vi "StudentScope - Calculate Cursor Values.vi"(5 "Scope graph":refnum<vi>, 6 "C2 Select":u32, 7 "C1 Select":u32, 8 "Array":dbl[][](array[numeric]), 9 "Rate":dbl) -> (0 "C2 Voltage":string, 1 "dV":string, 2 "C1 Voltage":string, 3 "dT":string)   [LabVIEW 2015]
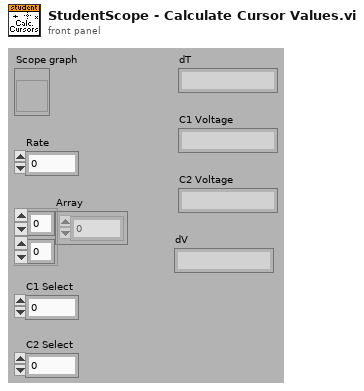
[diagram p1: front panel]
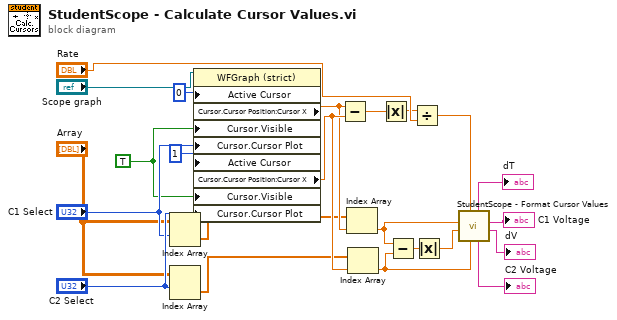
[diagram p0: block diagram]
diagram:
  w17 = TRUE ("Cursor.Visible")
  n1 = Index Array(array="Array", index (row)="C1 Select") -> (element=w11:dbl[])  [unwired: 1 in]
  n2 = Index Array(array="Array", index (row)="C2 Select") -> (element=w12:dbl[])  [unwired: 1 in]
  n3 = property class="WFGraph (strict)"(reference="Scope graph", "Active Cursor"=u32 0, "Cursor.Visible"=w17, "Cursor.Cursor Plot"="C1 Select", "Active Cursor"=u32 1, "Cursor.Visible"=w17, "Cursor.Cursor Plot"="C2 Select") -> ("Cursor.Cursor Position:Cursor X"=w19:dbl, "Cursor.Cursor Position:Cursor X"=w20:dbl)  [unwired: 1 in, 2 out]
  n4 = Subtract(x=w19, y=w20) -> (x-y=w6:dbl)
  n5 = Index Array(array=w11, index=w19) -> (element=w4:dbl)
  n6 = Index Array(array=w12, index=w20) -> (element=w5:dbl)
  n7 = Absolute Value(x=w6) -> (abs(x)=w13:dbl)
  n8 = Subtract(x=w4, y=w5) -> (x-y=w3:dbl)
  n9 = Divide(x=w13, y="Rate") -> (x/y=w14:dbl)
  n10 = Absolute Value(x=w3) -> (abs(x)=w2:dbl)
  n11 = call "StudentScope - Format Cursor Values.vi"("C2 Voltage In"=w5, "dT In"=w14, "dV In"=w2, "C1 Voltage In"=w4) -> ("dV"=→"dV":string, "C1 Voltage"=→"C1 Voltage":string, "C2 Voltage"=→"C2 Voltage":string, "dT"=→"dT":string)  [unwired: 4 in]
